vi "Reset-lasing.vi"(8 "error in (no error)":errorcluster, 11 "Object ref in":T1) -> (0 "error out":errorcluster, 3 "Object ref out":T1)   [LabVIEW 2013, in "SLMControl.lvlib" / "SC-Main.lvclass"]
uses:
  SC-Main.lvclass
  Object-reference.ctl
  UI/Control-names.ctl
  SC-Main.lvclass/SC-Main.ctl
  Read Lasing control.vi
  Read UI.vi
  UI/Set-control-string.vi
  SM1000/SM1000.lvclass
  UI/SC-UI.lvclass
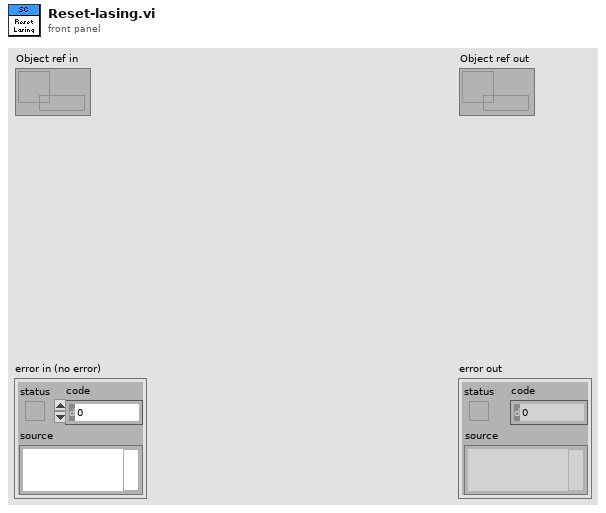
[diagram p1: front panel]
types:
  T1 = typedef "SLMControl.lvlib/SC-Main.lvclass/Object-reference.ctl" = refnum<data-value>
  T2 = typedef "SLMControl.lvlib/SC-UI.lvclass/Control-names.ctl" = enum16{"Com-in", "Com-out", "Help", "Status", "Load configuration", "Save configuration", "Load lasing files", "Load deposition files", "Clear", "Files", "Activate", "Execute", "Abort", "Options", "Current layer", "Current iteration", "Last elapsed time", "Deposition status", "Lasing job", "Status LEDs", "Exiting led", "Initialized led", "Files loaded led", "Activated led", "Executing led", "Deposition led", "Lasing job led", "Lasing led"}
  T3 = typedef "SLMControl.lvlib/SM1000.lvclass/Object-reference.ctl" = refnum<data-value>
  T4 = typedef "SLMControl.lvlib/SC-UI.lvclass/Panes-reference.ctl" = refnum<data-value>
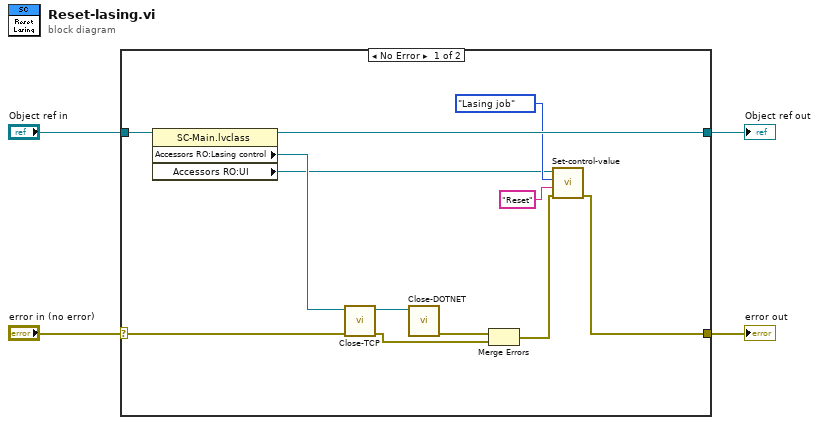
[diagram p0: block diagram]
diagram:
  n1 = case shown="No Error" "error in (no error)" {
    selector: "error in (no error)" -> [w14 w18]
    tunnel: [w6 w18] -> w3
    tunnel: [w15 w17] -> w1
    tunnel: "Object ref in" -> [w16 w17]
    frame No Error {
      n2 = property class="SC-Main.lvclass"(reference=w16) -> (reference out=w15:T1, "Accessors RO:Lasing control"=w12:T3, "Accessors RO:UI"=w8:T4)  [unwired: 1 in, 1 out]
      n3 = call "Close-TCP.vi"("error in (no error)"=w14, "SM1000-control in"=w12) -> ("error out"=w11:errorcluster, "SM1000-control out"=w5:T3)  [unwired: 7 in, 1 out]
      n4 = call "Close-DOTNET.vi"("SM1000-control in"=w5) -> ("error out"=w13:errorcluster)  [unwired: 8 in, 2 out]
      n5 = Merge Errors(w13, w11) -> (w7:errorcluster)
      n6 = call-poly "Set-control-value.vi"("error in (no error)"=w7, "Value"="Reset", "Control name"=Control-names."Lasing job", "Panes in"=w8) -> ("error out"=w6:errorcluster)  [unwired: 6 in, 1 out]
    }
    frame Error {
    }
  }
  "error out" <- w3
  "Object ref out" <- w1
